vi "10_NOV_FINAL.vi"() -> ()   [LabVIEW 2020]
uses:
  <instrlib>/Agilent B2900 Series/Agilent B2900 Series.lvlib
panel:
  in  "stop":bool
  out "Voltage":dbl(graph)
  out "Current":dbl(graph)
  out "XY Graph":cluster{"X":dbl[], "Y":dbl[]}[](graph)
  out "Current (Ampere)":dbl
  out "Resistance (Ohms)":dbl
  out "Voltage (Volt)":dbl
  in  "SELECT DEVICE":refnum<visa-resource-name>="USB0::0x0957::0x8E18::MY51140695::INSTR"
  in  "Source Voltage(V)":dbl
  in  "Channel":enum16{"Not Selected", "1", "2"}(ring)
  # "Select Values"
  # "Measured Values"
  # "Y"
  # "X"
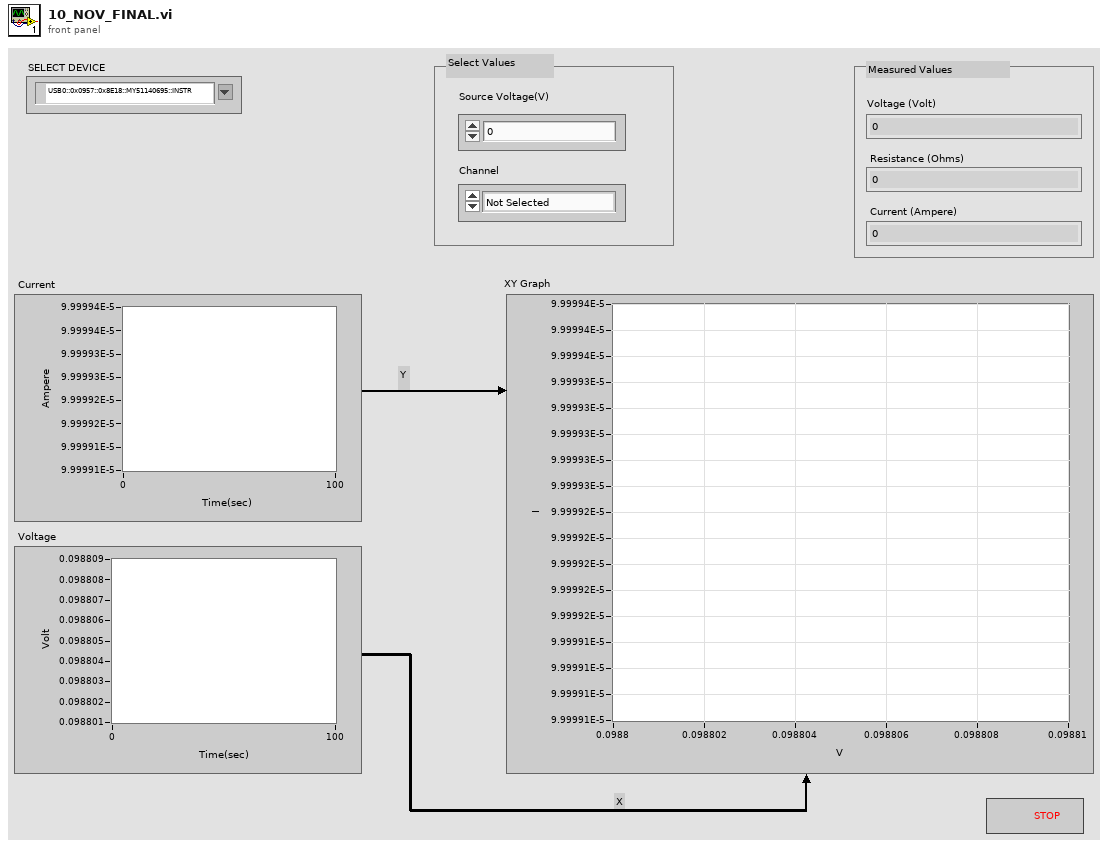
[diagram p1: front panel]
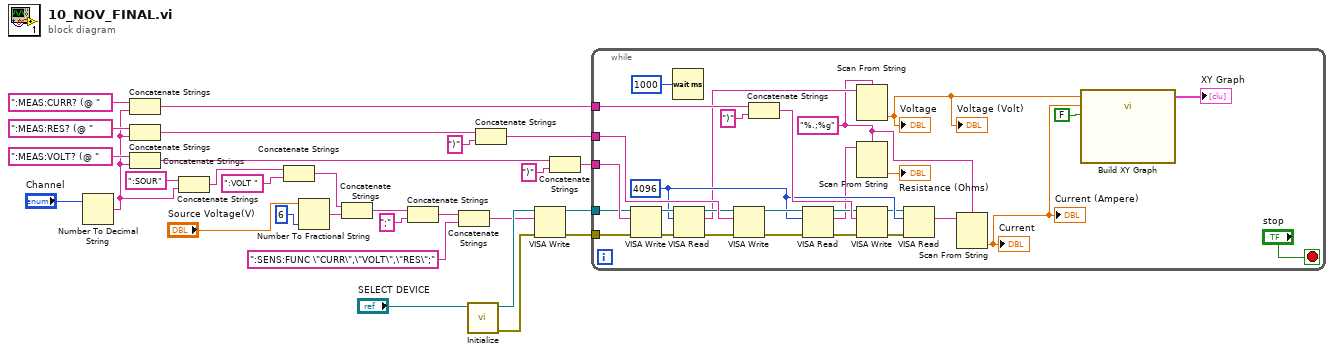
[diagram p0: block diagram]
diagram:
  n1 = Number To Decimal String(number="Channel") -> (decimal integer string=w3:string)  [unwired: 1 in]
  n2 = Concatenate Strings(":MEAS:CURR? (@ " ("string"), w3) -> (w9:string)
  n3 = Concatenate Strings(":MEAS:RES? (@ " ("string"), w3) -> (w7:string)
  n4 = Concatenate Strings(":MEAS:VOLT? (@ " ("string"), w3) -> (w13:string)
  n5 = Concatenate Strings(":SOUR", w3) -> (w28:string)
  n6 = Concatenate Strings(w28, ":VOLT ") -> (w26:string)
  n7 = Number To Fractional String(number="Source Voltage(V)", precision (6)=i16 6) -> (F-format string=w21:string)  [unwired: 2 in]
  n8 = Concatenate Strings(w26, w21) -> (w25:string)
  n9 = Concatenate Strings(w25, ";" ("string")) -> (w20:string)
  n10 = Concatenate Strings(w20, ":SENS:FUNC \"CURR\",\"VOLT\",\"RES\";") -> (w14:string)
  n11 = call <instrlib>:"Initialize.vi"("VISA resource name"="SELECT DEVICE") -> ("error out"=w15:errorcluster, "VISA resource name out"=w16:refnum<visa-resource-name>)  [unwired: 9 in]
  n12 = Concatenate Strings(w7, ")" ("string")) -> (w4:string)
  n13 = VISA Write(VISA resource name=w16, write buffer=w14, error in (no error)=w15) -> (VISA resource name out=w1:refnum<visa-resource-name>, error out=w2:errorcluster)  [unwired: 1 out]
  n14 = Concatenate Strings(w13, ")" ("string")) -> (w10:string)
  n15 = while {
    tunnel: w10 -> [w58]
    tunnel: w9 -> [w57]
    tunnel: w4 -> [w54]
    tunnel: w2 -> [w48]
    tunnel: w1 -> [w41]
    stop <- "stop" stop-if-true
    w30 = "%.;%g" ("format string")
    w49 = u32 4096 ("byte count")
    n16 = VISA Write(VISA resource name=w41, write buffer=w58, error in (no error)=w48) -> (VISA resource name out=w53:refnum<visa-resource-name>, error out=w52:errorcluster)  [unwired: 1 out]
    n17 = Wait (ms)(milliseconds to wait=u32 1000) -> ()  [unwired: 1 out]
    n18 = VISA Read(VISA resource name=w53, byte count=w49, error in (no error)=w52) -> (VISA resource name out=w47:refnum<visa-resource-name>, read buffer=w37:string, error out=w46:errorcluster)  [unwired: 1 out]
    n19 = VISA Write(VISA resource name=w47, write buffer=w54, error in (no error)=w46) -> (VISA resource name out=w51:refnum<visa-resource-name>, error out=w50:errorcluster)  [unwired: 1 out]
    n20 = Concatenate Strings(w57, ")" ("string")) -> (w55:string)
    n21 = VISA Read(VISA resource name=w51, byte count=w49, error in (no error)=w50) -> (VISA resource name out=w45:refnum<visa-resource-name>, read buffer=w40:string, error out=w44:errorcluster)  [unwired: 1 out]
    n22 = Scan From String(format string=w30, input string=w37) -> (output 1=w33:dbl)  [unwired: 3 in, 3 out]
    "Voltage (Volt)" <- w33
    "Voltage" <- w33
    n23 = Scan From String(format string=w30, input string=w40) -> (output 1=→"Resistance (Ohms)":dbl)  [unwired: 3 in, 3 out]
    n24 = VISA Write(VISA resource name=w45, write buffer=w55, error in (no error)=w44) -> (VISA resource name out=w43:refnum<visa-resource-name>, error out=w42:errorcluster)  [unwired: 1 out]
    n25 = VISA Read(VISA resource name=w43, byte count=w49, error in (no error)=w42) -> (read buffer=w39:string)  [unwired: 3 out]
    n26 = Scan From String(format string=w30, input string=w39) -> (output 1=w34:dbl)  [unwired: 3 in, 3 out]
    "Current (Ampere)" <- w34
    "Current" <- w34
    n27 = call "Build XY Graph"("Reset"=FALSE, "Y Input"=w34, "X Input"=w33) -> ("XY Graph"=→"XY Graph":cluster{"X":dbl[], "Y":dbl[]}[])  [unwired: 7 in, 1 out]
  }
